vi "ElevatorSim_example.vi"() -> ()   [LabVIEW 2019]
uses:
  <vilib>/Rock Robotics/WPI/ThirdParty/JAS_Junk/TrajLib/DCMOTOR.CTL
  <vilib>/Rock Robotics/WPI/ThirdParty/JAS_Junk/TrajLib/LINEAR_SYSTEM.ctl
  <vilib>/Analysis/Matrix/Datatypes/RealMatrix.ctl
  <vilib>/Rock Robotics/WPI/ThirdParty/JAS_Junk/TrajLib/LINEAR_QUADRATIC_REGULATOR.ctl
  <vilib>/Rock Robotics/WPI/ThirdParty/JAS_Junk/TrajLib/KALMAN_FILTER.ctl
  <vilib>/Rock Robotics/WPI/ThirdParty/JAS_Junk/TrajLib/LINEAR_SYSTEM_LOOP.ctl
  <vilib>/Rock Robotics/WPI/ThirdParty/JAS_Junk/TrajLib/LINEAR_PLANT_INV_FF.ctl
  <vilib>/Rock Robotics/WPI/ThirdParty/JAS_Junk/TrajLib/ELEVATOR_SIM.ctl
  <vilib>/Rock Robotics/WPI/ThirdParty/JAS_Junk/TrajLib/LINEAR_SYSTEM_SIM.ctl
  <vilib>/Rock Robotics/WPI/ThirdParty/JAS_Junk/TrajLib/MatBuilder_Create.vi
  <vilib>/Rock Robotics/WPI/ThirdParty/JAS_Junk/TrajLib/DCMotor_New.vi
  <vilib>/Rock Robotics/WPI/ThirdParty/JAS_Junk/TrajLib/Units_RotationsPerMinuteToRadiansPerSecond.vi
  <vilib>/Rock Robotics/WPI/ThirdParty/JAS_Junk/TrajLib/LinearSystem_New.vi
  <vilib>/Rock Robotics/WPI/ThirdParty/JAS_Junk/TrajLib/MatBuilder_Fill.vi
  <vilib>/Rock Robotics/WPI/ThirdParty/JAS_Junk/TrajLib/MatrixHelper_Zero.vi
  <vilib>/Rock Robotics/WPI/ThirdParty/JAS_Junk/TrajLib/MatrixHelper_CoerceSize.vi
  <vilib>/Rock Robotics/WPI/ThirdParty/JAS_Junk/TrajLib/Trajectory_Library.lvlib
  <vilib>/Analysis/Matrix/NI_Matrix.lvlib
panel:
  in  "Tab Control":T1(tab)
  out "Battery Voltage":dbl format="%20.3f"
  out "CO Chart":cluster{dbl, "Voltage":dbl}(graph)
  in  "GO UP":bool
  out "Elevator\nHeight":dbl(slide) scale=-1.0..6.0
  out "Height":dbl format="%20.3f"
  out "Cor Err":bool
  out "Kalman Filtered\nHeight":dbl format="%20.3f"
  out "PV Chart":T2(graph)
  out "Predict Err":bool
  out "Motor Volt Dmd (CO)":dbl format="%20.3f"
  out "At Top":bool
  out "At Bottom":bool
  out "Motor Amps":dbl format="%20.3f"
  out "Elevator Motor":T3 {"Jr_KgM2" format="%13.5p"; "L_H" format="%13.5p"; "Kt_NMPerAmp" format="%13.5p"; "KvINV_RadPerSecPerVolt" format="%13.5p"; "R_Ohms" format="%13.5p"; "FreeSpeed_RadPerSec" format="%13.5p"; "FreeCurrent_Amps" format="%13.5p"; "StallCurrent_Amps" format="%13.5p"; "StallTorque_NM" format="%13.5p"; "nominalVoltage_Volts" format="%13.5p"}
  out "m_Elevator":T4
  out "Elevator Simulaation":T6 {"GearBox"."Jr_KgM2" format="%13.5p"; "GearBox"."L_H" format="%13.5p"; "GearBox"."Kt_NMPerAmp" format="%13.5p"; "GearBox"."KvINV_RadPerSecPerVolt" format="%13.5p"; "GearBox"."R_Ohms" format="%13.5p"; "GearBox"."FreeSpeed_RadPerSec" format="%13.5p"; "GearBox"."FreeCurrent_Amps" format="%13.5p"; "GearBox"."StallCurrent_Amps" format="%13.5p"; "GearBox"."StallTorque_NM" format="%13.5p"; "GearBox"."nominalVoltage_Volts" format="%13.5p"}
  out "KalmanFilter":T8
  out "Kalman Error":errorcluster
  out "LinearQuadraticRegulator":T9
  out "LQR Error":bool
  out "Linear System Loop":T10
  out "LinSysLoop_Error":bool
  # "<States,States>"
  # "<States,Inputs>"
  # "<Outputs,States>"
  # "<Outputs,Inputs>"
  # "<States, 1>"
  # "<Outputs, 1>"
  # "<Inputs, 1>"
  # "<Outputs, 1>"
  # "<States,States>"
  # "<States,Inputs>"
  # "<Outputs,States>"
  # "<Outputs,Inputs>"
  # "Steady State Gain  \n<States,Outputs>"
  # "State Estimate <Statess,1>"
  # "<States,States>"
  # "<States,Inputs>"
  # "<Outputs,States>"
  # "<Outputs,Inputs>"
  # "Ref State <States,1>"
  # "Comp and capped \noutput <Inputs,1>"
  # "Controller gain\n<Inputs,States>"
  # "<States,1>"
  # "<FUTURE --- CLAMP TYPE -- For now\nuse Normalize>"
  # "Steady State Gain  \n<States,Outputs>"
  # "State Estimate <Statess,1>"
  # "<States,States>"
  # "<States,Inputs>"
  # "<Outputs,States>"
  # "<Outputs,Inputs>"
  # "<States,1>"
  # "<Inputs,1>"
  # "<States,Inputs>"
  # "<States,States>"
  # "Ref State <States,1>"
  # "Comp and capped \noutput <Inputs,1>"
  # "Controller gain\n<Inputs,States>"
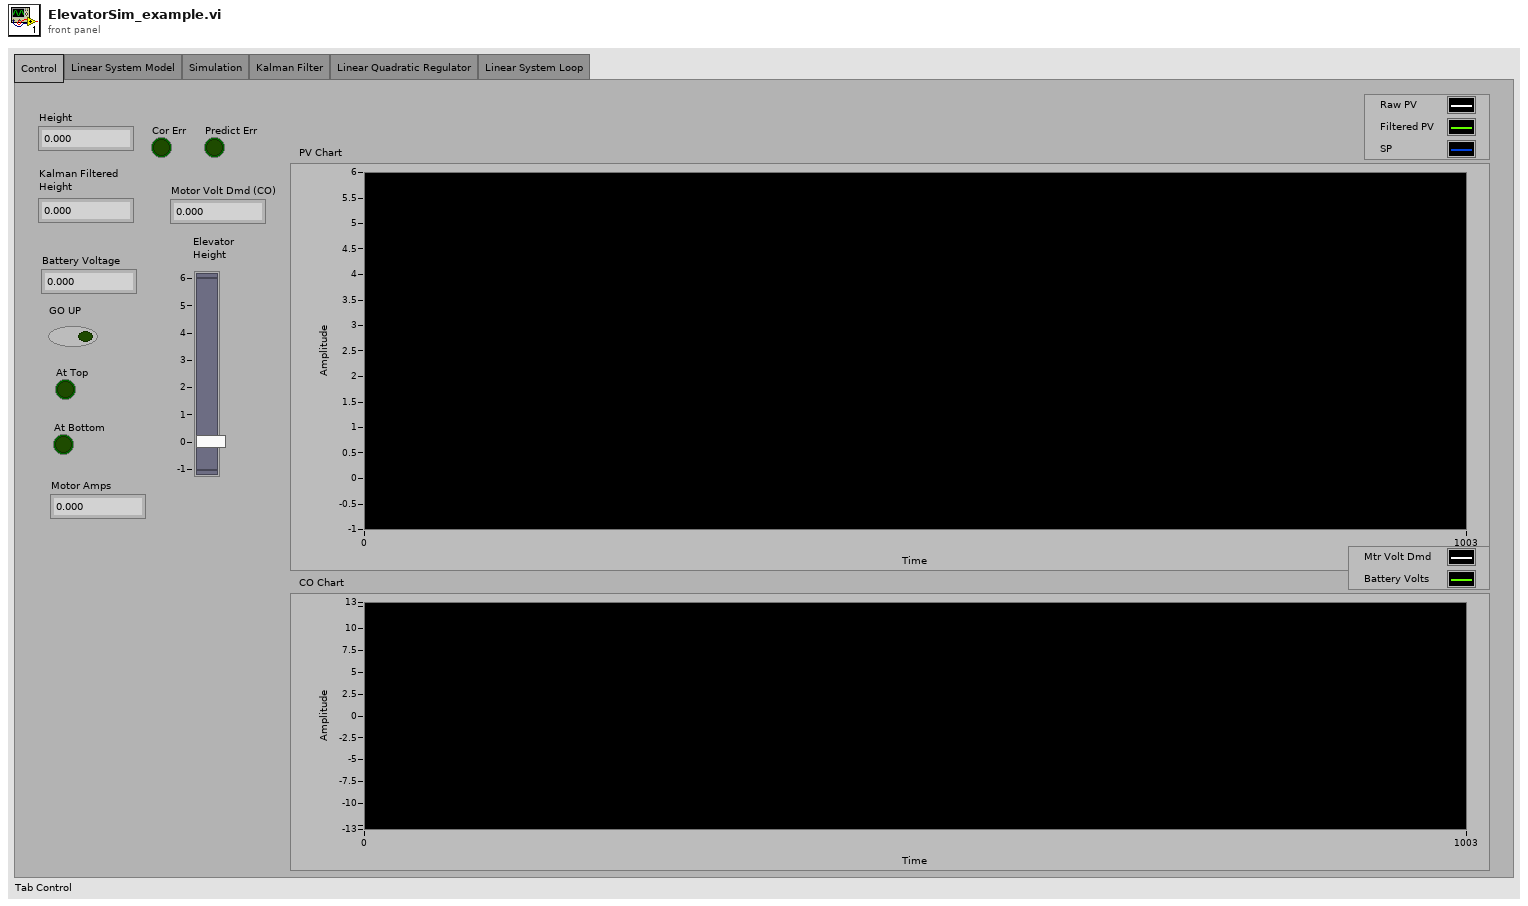
[diagram p1: front panel]
types:
  T1 = enum32{"Control", "Linear System Model", "Simulation", "Kalman Filter", "Linear Quadratic Regulator", "Linear System Loop"}
  T2 = cluster{"upper limit":dbl, "Real Matrix Element":dbl, "Real Matrix Element":dbl}
  T3 = typedef "Trajectory_Library.lvlib/DCMOTOR.CTL" = cluster{"nominalVoltage_Volts":dbl, "StallTorque_NM":dbl, "StallCurrent_Amps":dbl, "FreeCurrent_Amps":dbl, "FreeSpeed_RadPerSec":dbl, "R_Ohms":dbl, "KvINV_RadPerSecPerVolt":dbl, "Kt_NMPerAmp":dbl, "L_H":dbl, "Jr_KgM2":dbl}
  T4 = typedef "Trajectory_Library.lvlib/LINEAR_SYSTEM.ctl" = cluster{"m_A":T5, "m_B":T5, "m_C":T5, "m_D":T5, "States":i32, "Inputs":i32, "Outputs":i32}
  T5 = typedef "NI_Matrix.lvlib/RealMatrix.ctl" = dbl[][]
  T6 = typedef "Trajectory_Library.lvlib/ELEVATOR_SIM.ctl" = cluster{"LinearSystemSim":T7, "GearBox":T3, "Gearing":dbl, "DrumRadius_M":dbl, "MinHeight_M":dbl, "MaxHeight_M":dbl, "CarriageMass_Kg":dbl}
  T7 = typedef "Trajectory_Library.lvlib/LINEAR_SYSTEM_SIM.ctl" = cluster{"m_Plant":T4, "m_X":T5, "m_Y":T5, "m_U":T5, "MeasureStdDev":T5}
  T8 = typedef "Trajectory_Library.lvlib/KALMAN_FILTER.ctl" = cluster{"m_K":T5, "m_xHat":T5, "States":i32, "Outputs":i32, "m_Plant":T4}
  T9 = typedef "Trajectory_Library.lvlib/LINEAR_QUADRATIC_REGULATOR.ctl" = cluster{"m_r":T5, "m_U":T5, "m_K":T5, "States":i32, "Inputs":i32}
  T10 = typedef "Trajectory_Library.lvlib/LINEAR_SYSTEM_LOOP.ctl" = cluster{"Controller":T9, "FeedForward":T11, "Observer":T8, "Next_R":T5, "Clamp Max":T5}
  T11 = typedef "Trajectory_Library.lvlib/LINEAR_PLANT_INV_FF.ctl" = cluster{"m_R":T5, "m_Uff":T5, "m_B":T5, "m_A":T5, "States":i32, "Inputs":i32}
  T12 = cluster{"Position_Meters":dbl, "Real Matrix Element":dbl, "Real Matrix Element":dbl}
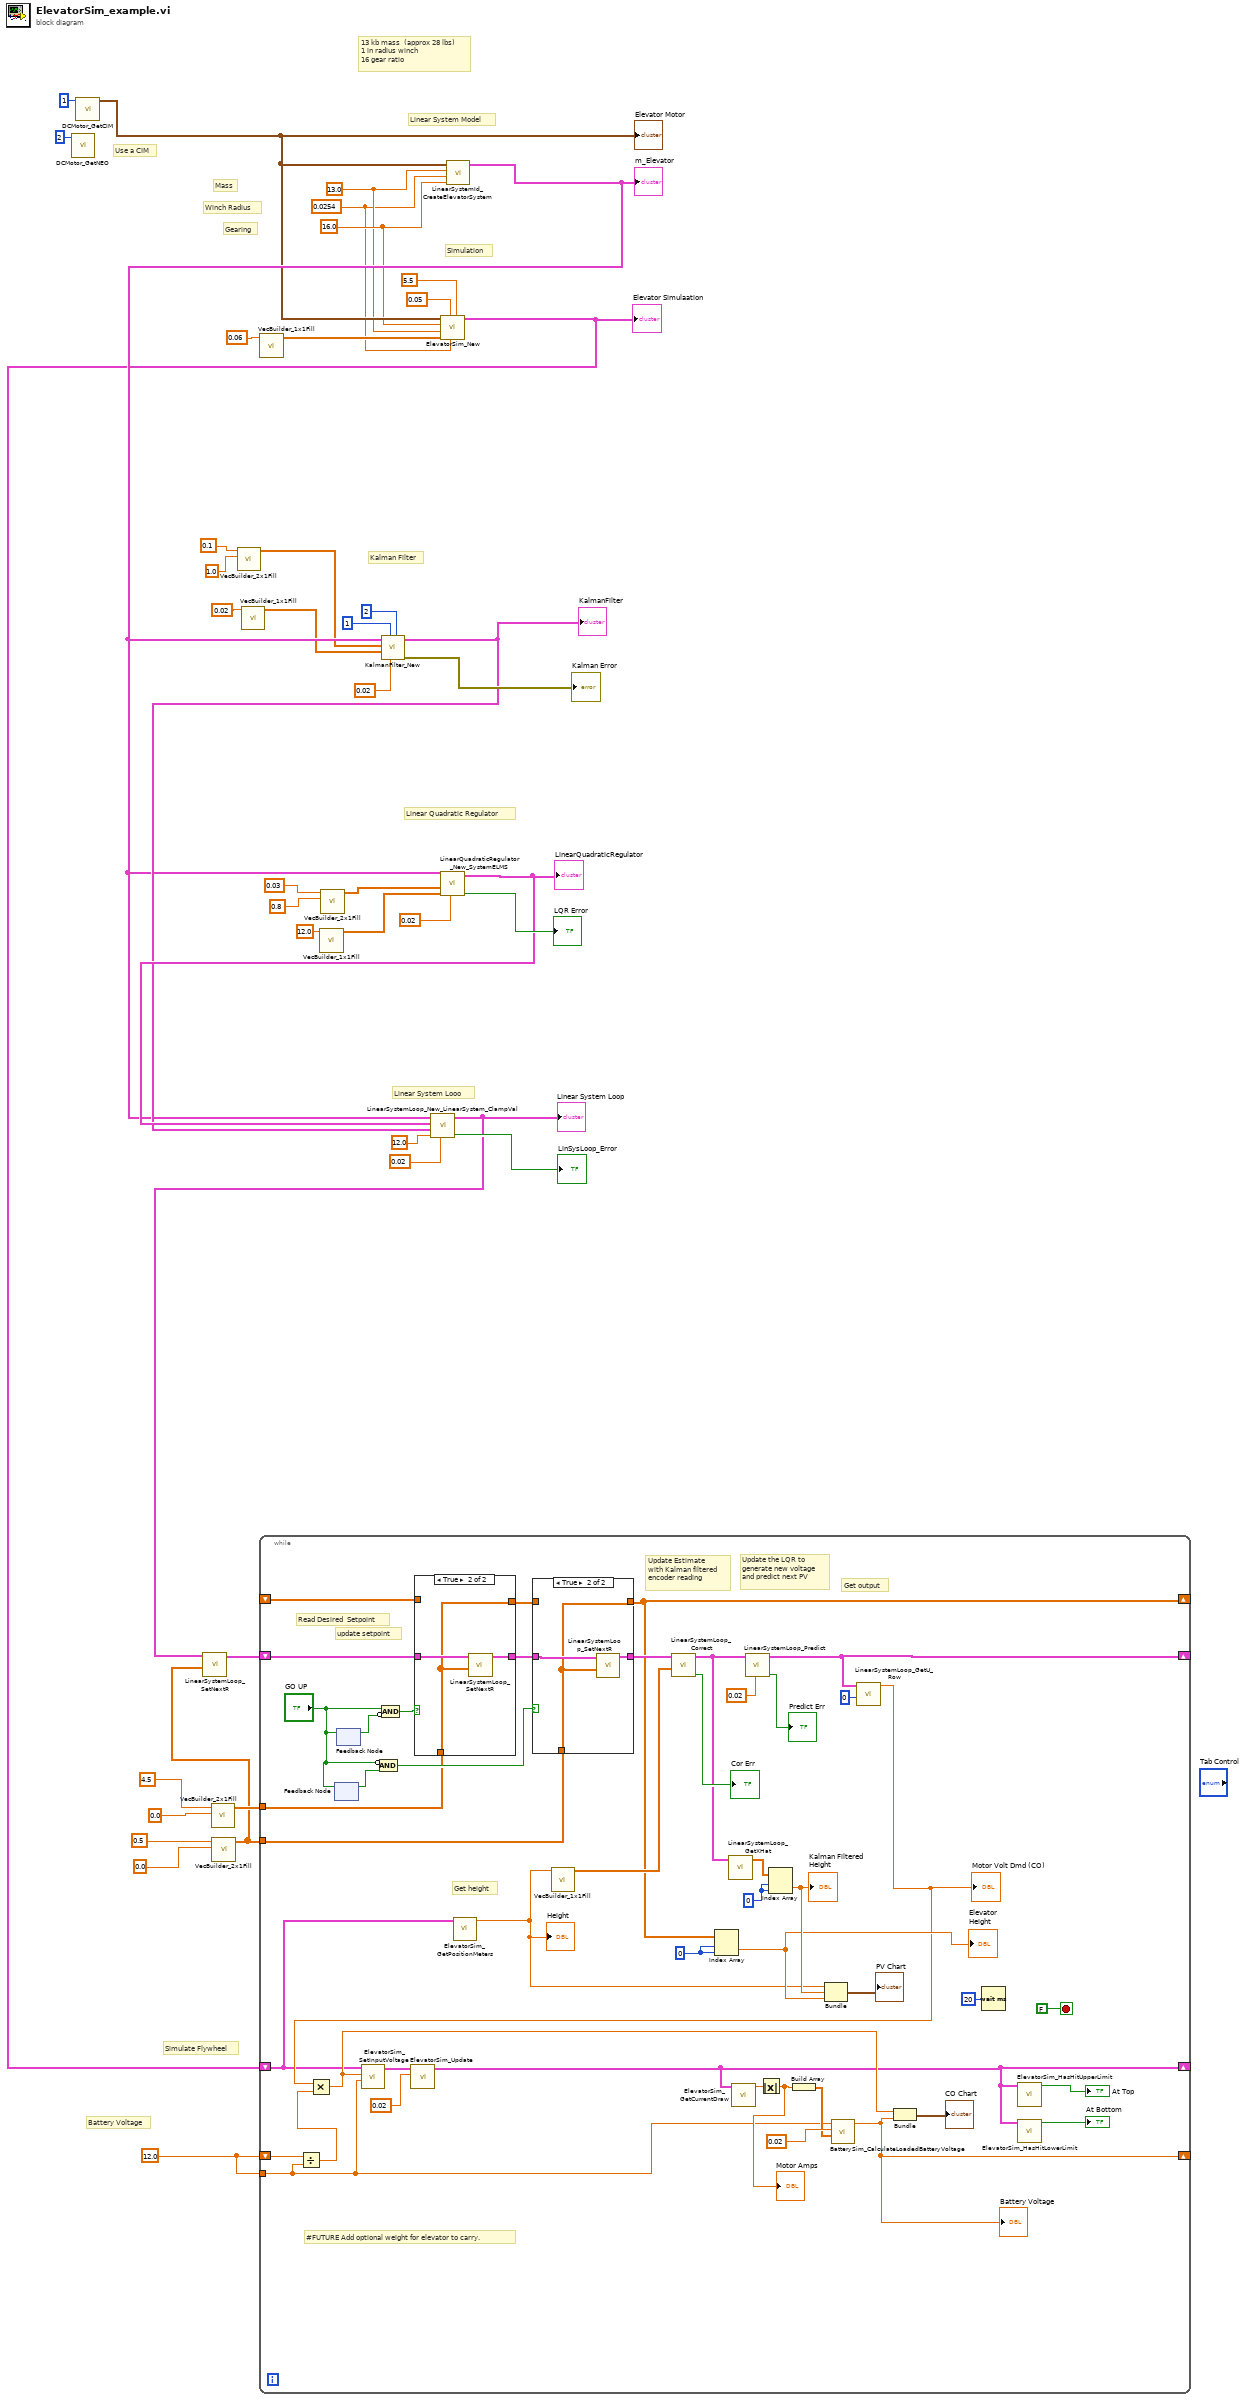
[diagram p0: block diagram]
diagram:
  w26 = 16.0 ("G")
  w24 = 0.0254 ("radiusMeters")
  w25 = 13.0 ("massKg")
  w34 = 12.0
  # "Linear System Looo"
  # "Linear Quadratic Regulator"
  # "Kalman Filter"
  # "Simulation"
  # "Linear System Model"
  # "Mass"
  # "Winch Radius"
  # "Simulate Flywheel"
  # "13 kb mass  (approx 28 lbs)\n1 in radius winch\n16 gear ratio"
  # "Gearing"
  # "Use a CIM"
  # "Battery Voltage"
  n1 = call <vilib>:"DCMotor_GetNEO.vi"("Num Motors"=2) -> ()  [unwired: 10 in, 1 out]
  n2 = call <vilib>:"DCMotor_GetCIM.vi"("Num Motors"=1) -> ("DCMOTOR"=w31:T3)  [unwired: 10 in]
  "Elevator Motor" <- w31
  n3 = call <vilib>:"VecBuilder_2x1Fill.vi"("R1"=0.0, "R0"=4.5 ("RotationsPerMinute")) -> ("output matrix"=w6:T5)  [unwired: 9 in]
  n4 = call <vilib>:"VecBuilder_2x1Fill.vi"("R1"=0.0, "R0"=0.5 ("R0_C0")) -> ("output matrix"=w1:T5)  [unwired: 9 in]
  n5 = call <vilib>:"VecBuilder_2x1Fill.vi"("R1"=1.0, "R0"=0.1 ("R0_C0")) -> ("output matrix"=w17:T5)  [unwired: 9 in]
  n6 = call <vilib>:"VecBuilder_1x1Fill.vi"("R0_C0"=0.02) -> ("output matrix"=w16:T5)  [unwired: 10 in]
  n7 = call <vilib>:"VecBuilder_1x1Fill.vi"("R0_C0"=0.06) -> ("output matrix"=w27:T5)  [unwired: 10 in]
  n8 = call <vilib>:"VecBuilder_1x1Fill.vi"("R0_C0"=12.0) -> ("output matrix"=w10:T5)  [unwired: 10 in]
  n9 = call <vilib>:"VecBuilder_2x1Fill.vi"("R1"=0.8 ("R0_C0"), "R0"=0.03 ("R0_C0")) -> ("output matrix"=w12:T5)  [unwired: 9 in]
  n10 = call <vilib>:"ElevatorSim_New.vi"("MaxHeight_Meters"=5.5, "DrumRadius_Meters"=w24, "MinHeight_Meters"=0.05, "MeasurementStdDev"=w27, "CarriageMass_Kg"=w25, "Gearing"=w26, "GearBox"=w31) -> ("ElevatorSim"=w30:T6)  [unwired: 3 in, 1 out]
  "Elevator Simulaation" <- w30
  n11 = call <vilib>:"LinearSystemId_CreateElevatorSystem.vi"("G"=w26, "radiusMeters"=w24, "massKg"=w25, "DCMOTOR"=w31) -> ("Linearsystem"=w32:T4)  [unwired: 6 in, 1 out]
  "m_Elevator" <- w32
  n12 = call <vilib>:"KalmanFilter_New.vi"("States"=2, "dt_Seconds"=0.02, "Outputs"=1, "MeasurementStdDevs"=w16, "StateStdDevs"=w17, "Plant"=w32) -> ("Error"=→"Kalman Error":errorcluster, "KalmanFilter"=w38:T8)  [unwired: 4 in]
  "KalmanFilter" <- w38
  n13 = call <vilib>:"LinearQuadraticRegulator_New_SystemELMS.vi"("dt_Seconds"=0.02, "Relms"=w10, "Qelms"=w12, "LINEARSYSTEM"=w32) -> ("Error"=→"LQR Error":bool, "LinearQuadraticRegulator"=w39:T9)  [unwired: 6 in]
  "LinearQuadraticRegulator" <- w39
  n14 = call <vilib>:"LinearSystemLoop_New_LinearSystem_ClampVal.vi"("dT_Seconds"=0.02, "Max_Voltage"=12.0, "Observer"=w38, "Controller"=w39, "Plant"=w32) -> ("Error"=→"LinSysLoop_Error":bool, "Linear System Loop"=w2:T10)  [unwired: 5 in]
  "Linear System Loop" <- w2
  n15 = call <vilib>:"LinearSystemLoop_SetNextR.vi"("R"=w1, "input inear System Loop"=w2) -> ("out Linear System Loop"=w3:T10)  [unwired: 8 in, 1 out]
  n16 = while {
    shift-right: [w51] -> _
    shift-left: w3 -> [w81]
    tunnel: w6 -> [w79]
    tunnel: w1 -> [w78]
    shift-right: [w50] -> _
    shift-left: w30 -> [w45]
    shift-right: [w62] -> _
    shift-left: _ -> [w63]
    shift-right: [w53] -> _
    shift-left: w34 -> [w59]
    tunnel: w34 -> [w43]
    stop <- FALSE stop-if-true
    w61 = 0 ("index (row)")
    w74 = 0 ("index (row)")
    # "Get height"
    # "#FUTURE Add optional weight for elevator to carry."
    # "Get output"
    # "Update the LQR to \ngenerate new voltage\nand predict next PV"
    # "update setpoint"
    # "Read Desired  Setpoint"
    # "Update Estimate\nwith Kalman filtered\nencoder reading"
    n17 = Divide(x=w59, y=w43) -> (x/y=w57:dbl)
    n18 = feedback #1() -> (w85:bool)  [unwired: 1 in]
    n19 = feedback-in #1("GO UP") -> ()
    n20 = feedback-in #2("GO UP") -> ()
    n21 = feedback #2() -> (w86:bool)  [unwired: 1 in]
    n22 = Compound Arithmetic op=AND(invert "GO UP", w85) -> (w82:bool)
    n23 = Compound Arithmetic op=AND("GO UP", invert w86) -> (w83:bool)
    n24 = case shown="True" w83 {
      tunnel: w81 -> [w95 w97]
      tunnel: [w95 w98] -> w80
      tunnel: w79 -> [_ w96]
      tunnel: [w94 w96] -> w64
      tunnel: w63 -> [w94 _]
      frame False {
      }
      frame True {
        n25 = call <vilib>:"LinearSystemLoop_SetNextR.vi"("R"=w96, "input inear System Loop"=w97) -> ("out Linear System Loop"=w98:T10)  [unwired: 8 in, 1 out]
      }
    }
    n26 = call <vilib>:"ElevatorSim_GetPositionMeters.vi"("ElevatorSim"=w45) -> ("Position_Meters"=w44:dbl)  [unwired: 10 in]
    "Height" <- w44
    n27 = case shown="True" w82 {
      tunnel: w80 -> [w90 w92]
      tunnel: [w90 w93] -> w77
      tunnel: w78 -> [_ w91]
      tunnel: w64 -> [w89 _]
      tunnel: [w89 w91] -> w62
      frame False {
      }
      frame True {
        n28 = call <vilib>:"LinearSystemLoop_SetNextR.vi"("R"=w91, "input inear System Loop"=w92) -> ("out Linear System Loop"=w93:T10)  [unwired: 8 in, 1 out]
      }
    }
    n29 = call <vilib>:"VecBuilder_1x1Fill.vi"("R0_C0"=w44) -> ("output matrix"=w76:T5)  [unwired: 10 in]
    n30 = call <vilib>:"LinearSystemLoop_Correct.vi"("Y"=w76, "input inear System Loop"=w77) -> ("Error"=→"Cor Err":bool, "out Linear System Loop"=w70:T10)  [unwired: 8 in]
    n31 = Index Array(array=w62, index (row)=w61, index (col)=w61) -> (element=w60:dbl)
    "Elevator\nHeight" <- w60
    n32 = call <vilib>:"LinearSystemLoop_GetXHat.vi"("input inear System Loop"=w70) -> ("XHat"=w73:T5)  [unwired: 10 in]
    n33 = call <vilib>:"LinearSystemLoop_Predict.vi"("dT_Seconds"=0.02, "input inear System Loop"=w70) -> ("Error"=→"Predict Err":bool, "out Linear System Loop"=w51:T10)  [unwired: 8 in]
    n34 = Index Array(array=w73, index (row)=w74, index (col)=w74) -> (element=w72:dbl)
    "Kalman Filtered\nHeight" <- w72
    n35 = Bundle("Position_Meters"=w44, "Real Matrix Element"=w72, "Real Matrix Element"=w60) -> (→"PV Chart":T12)  [unwired: 1 in]
    n36 = call <vilib>:"LinearSystemLoop_GetU_Row.vi"("Row"=0, "input inear System Loop"=w51) -> ("U"=w58:dbl)  [unwired: 9 in]
    "Motor Volt Dmd (CO)" <- w58
    n37 = Multiply(x=w58, y=w57) -> (x*y=w52:dbl)
    n38 = call <vilib>:"ElevatorSim_SetInputVoltage.vi"("Battery_Volts"=w43, "Input_Voltage"=w52, "in ElevatorSim"=w45) -> ("out ElevatorSim"=w66:T6)  [unwired: 8 in]
    n39 = call <vilib>:"ElevatorSim_Update.vi"("dT_Seconds"=0.02, "in ElevatorSim"=w66) -> ("out ElevatorSim"=w50:T6)  [unwired: 8 in, 1 out]
    n40 = call <vilib>:"ElevatorSim_GetCurrentDraw.vi"("ElevatorSim"=w50) -> ("Current_Amps"=w47:dbl)  [unwired: 10 in]
    n41 = Absolute Value(x=w47) -> (abs(x)=w46:dbl)
    "Motor Amps" <- w46
    n42 = Build Array(w46) -> (w55:dbl[])
    n43 = call <vilib>:"BatterySim_CalculateLoadedBatteryVoltage.vi"("Currents"=w55, "Resistance_Ohms"=0.02, "NominalVoltage"=w43) -> ("Voltage"=w53:dbl)  [unwired: 8 in]
    "Battery Voltage" <- w53
    n44 = Bundle(w52, "Voltage"=w53) -> (→"CO Chart":cluster{dbl, "Voltage":dbl})  [unwired: 1 in]
    n45 = Wait (ms)(milliseconds to wait=u32 20) -> ()  [unwired: 1 out]
    n46 = call <vilib>:"ElevatorSim_HasHitUpperLimit.vi"("ElevatorSim"=w50) -> ("At HIgh LImit"=→"At Top":bool)  [unwired: 10 in]
    n47 = call <vilib>:"ElevatorSim_HasHitLowerLimit.vi"("ElevatorSim"=w50) -> ("AtLowLimit"=→"At Bottom":bool)  [unwired: 10 in]
  }
